vi "Convert Array to image.vi"() -> ()   [LabVIEW 2014]
uses:
  <vilib>/Utility/file.llb/Read From Spreadsheet File (DBL).vi
panel:
  out "Image Out 2":T1(plugin-control)
  out "Picture":picture
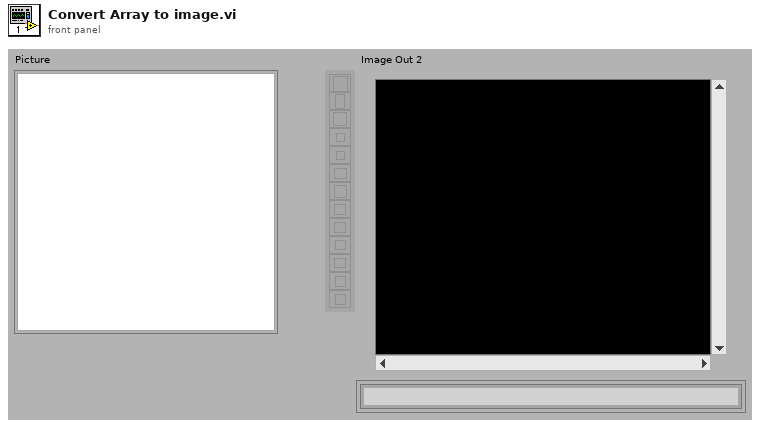
[diagram p1: front panel]
types:
  T1 = typedef "IMAQ Image.ctl" = refnum<image>
  T2 = typedef "imagedata.ctl" = cluster{"image type":i32, "image depth":i32, "image":u8[], "mask":u8[], "colors":u32[], "Rectangle":cluster{"left":i16, "top":i16, "right":i16, "bottom":i16}}
  T3 = cluster{"Position":cluster{"X":sgl, "Y":sgl}, "Radius":dbl, "Score":dbl}[]
  T4 = cluster{"Corners":cluster{"X":sgl, "Y":sgl}[], "Orientation (degrees)":dbl, "Width":dbl, "Height":dbl, "Score":dbl}[]
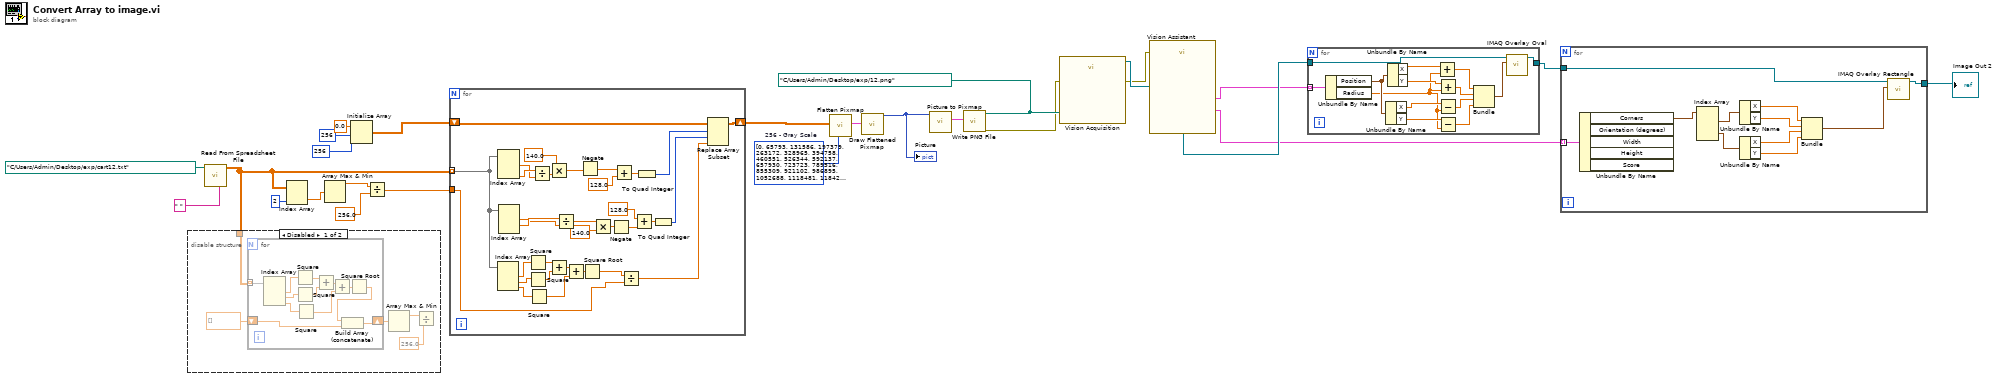
[diagram p0: block diagram]
diagram:
  w12 = path "C:/Users/Admin/Desktop/exp/12.png" ("path to PNG file")
  w15 = u32[] [0, 65793, 131586, 197379, 263172, 328965, 394758, 460551, 526344, 592137, 657930, 723723, 789516, 855309, 921102, 986895, 1052688, 1118481, 1184274, 1250067, 1315860, 1381653, 1447446, 1513239, 1579032, 1644825, 1710618, 1776411, 1842204, 1907997, 1973790, 2039583, 2105376, 2171169, 2236962, 2302755, 2368548, 2434341, 2500134, 2565927, 2631720, 2697513, 2763306, 2829099, 2894892, 2960685, 3026478, 3092271, 3158064, 3223857, 3289650, 3355443, 3421236, 3487029, 3552822, 3618615, 3684408, 3750201, 3815994, 3881787, 3947580, 4013373, 4079166, 4144959, 4210752, 4276545, 4342338, 4408131, 4473924, 4539717, 4605510, 4671303, 4737096, 4802889, 4868682, 4934475, 5000268, 5066061, 5131854, 5197647, 5263440, 5329233, 5395026, 5460819, 5526612, 5592405, 5658198, 5723991, 5789784, 5855577, 5921370, 5987163, 6052956, 6118749, 6184542, 6250335, 6316128, 6381921, 6447714, 6513507, 6579300, 6645093, 6710886, 6776679, 6842472, 6908265, 6974058, 7039851, 7105644, 7171437, 7237230, 7303023, 7368816, 7434609, 7500402, 7566195, 7631988, 7697781, 7763574, 7829367, 7895160, 7960953, 8026746, 8092539, 8158332, 8224125, 8289918, 8355711, 8421504, 8487297, 8553090, 8618883, 8684676, 8750469, 8816262, 8882055, 8947848, 9013641, 9079434, 9145227, 9211020, 9276813, 9342606, 9408399, 9474192, 9539985, 9605778, 9671571, 9737364, 9803157, 9868950, 9934743, 10000536, 10066329, 10132122, 10197915, 10263708, 10329501, 10395294, 10461087, 10526880, 10592673, 10658466, 10724259, 10790052, 10855845, 10921638, 10987431, 11053224, 11119017, 11184810, 11250603, 11316396, 11382189, 11447982, 11513775, 11579568, 11645361, 11711154, 11776947, 11842740, 11908533, 11974326, 12040119, 12105912, 12171705, 12237498, 12303291, 12369084, 12434877, 12500670, 12566463, 12632256, 12698049, 12763842, 12829635, 12895428, 12961221, 13027014, 13092807, 13158600, 13224393, 13290186, 13355979, 13421772, 13487565, 13553358, 13619151, 13684944, 13750737, 13816530, 13882323, 13948116, 14013909, 14079702, 14145495, 14211288, 14277081, 14342874, 14408667, 14474460, 14540253, 14606046, 14671839, 14737632, 14803425, 14869218, 14935011, 15000804, 15066597, 15132390, 15198183, 15263976, 15329769, 15395562, 15461355, 15527148, 15592941, 15658734, 15724527, 15790320, 15856113, 15921906, 15987699, 16053492, 16119285, 16185078, 16250871, 16316664, 16382457, 16448250, 16514043, 16579836, 16645629, 16711422, 16777215]  # 256 - Gray Scale
  n1 = call-poly <vilib>:"Read From Spreadsheet File.vi"("delimiter (\\t)"=" " ("delimiter (\\t)"), "file path (dialog if empty)"=path "C:/Users/Admin/Desktop/exp/cart12.txt") -> ("all rows"=w4:dbl[][])  [unwired: 5 in, 4 out]
  n2 = disable-structure shown="Disabled" {
    disable-tunnel: w4 -> [w31 _]
    frame Disabled {
      n3 = for {
        tunnel: w31 -> [w35] mode=indexing
        shift-right: [w34] -> w27
        shift-left: dbl[] [] -> [w32]
        n4 = Index Array(array=w35) -> (element #1=w43:dbl, element #2=w42:dbl, element #3=w37:dbl)  [unwired: 3 in]
        n5 = Square(x=w43) -> (x^2=w41:dbl)
        n6 = Square(x=w42) -> (x^2=w40:dbl)
        n7 = Square(x=w37) -> (x^2=w36:dbl)
        n8 = Add(x=w41, y=w40) -> (x+y=w39:dbl)
        n9 = Add(x=w39, y=w36) -> (x+y=w38:dbl)
        n10 = Square Root(x=w38) -> (sqrt(x)=w33:dbl)
        n11 = Build Array (concatenate)(w33, w32) -> (w34:dbl[])
      }
      n12 = Array Max & Min(array=w27) -> (max value=w29:dbl)  [unwired: 3 out]
      n13 = Divide(x=w29, y=256.0) -> ()  [unwired: 1 out]
    }
    frame Enabled {
    }
  }
  n14 = Index Array(array=w4, index (col)=2 ("disabled index (col)")) -> (element=w19:dbl[])  [unwired: 1 in]
  n15 = Array Max & Min(array=w19) -> (max value=w18:dbl)  [unwired: 3 out]
  n16 = Initialize Array(0.0 ("element"), 256 ("dimension size"), 256 ("dimension size")) -> (w21:dbl[][])
  n17 = Divide(x=w18, y=256.0) -> (x/y=w3:dbl)
  n18 = for {
    tunnel: w4 -> [w69] mode=indexing
    shift-right: [w51] -> w16
    shift-left: w21 -> [w50]
    tunnel: w3 -> [w60]
    n19 = Index Array(array=w69) -> (element #1=w75:dbl, element #2=w74:dbl, element #3=w64:dbl)  [unwired: 3 in]
    n20 = Index Array(array=w69) -> (element #1=w56:dbl, element #3=w57:dbl)  [unwired: 3 in, 1 out]
    n21 = Index Array(array=w69) -> (element #1=w54:dbl, element #2=w55:dbl)  [unwired: 3 in, 1 out]
    n22 = Square(x=w75) -> (x^2=w73:dbl)
    n23 = Square(x=w74) -> (x^2=w72:dbl)
    n24 = Square(x=w64) -> (x^2=w63:dbl)
    n25 = Divide(x=w57, y=w56) -> (x/y=w67:dbl)
    n26 = Multiply(x=140.0, y=w67) -> (x*y=w47:dbl)
    n27 = Add(x=w73, y=w72) -> (x+y=w71:dbl)
    n28 = Divide(x=w55, y=w54) -> (x/y=w68:dbl)
    n29 = Add(x=w71, y=w63) -> (x+y=w70:dbl)
    n30 = Negate(x=w47) -> (-x=w46:dbl)
    n31 = Square Root(x=w70) -> (sqrt(x)=w61:dbl)
    n32 = Multiply(x=w68, y=140.0) -> (x*y=w45:dbl)
    n33 = Negate(x=w45) -> (-x=w44:dbl)
    n34 = Add(x=w46, y=128.0 ("x")) -> (x+y=w48:dbl)
    n35 = Divide(x=w61, y=w60) -> (x/y=w62:dbl)
    n36 = Add(x=128.0 ("y"), y=w44) -> (x+y=w49:dbl)
    n37 = To Quad Integer(1:w48) -> (0:w59:i64)
    n38 = To Quad Integer(1:w49) -> (0:w58:i64)
    n39 = Replace Array Subset(array=w50, new element=w62, index (row)=w59, index (col)=w58) -> (w51:dbl[][])
  }
  n40 = call <vilib>:"Flatten Pixmap.vi"("colors"=w15, "8-bit pixmap"=w16) -> ("image data"=w13:T2)  [unwired: 9 in]
  n41 = call <vilib>:"Draw Flattened Pixmap.vi"("image data"=w13) -> ("new picture"=w26:picture)  [unwired: 8 in]
  "Picture" <- w26
  n42 = call <vilib>:"Picture to Pixmap.vi"("picture"=w26) -> ("image data"=w14:T2)  [unwired: 9 in, 1 out]
  n43 = call <vilib>:"Write PNG File.vi"("image data"=w14, "path to PNG file"=w12) -> ("error out"=w2:errorcluster)  [unwired: 8 in, 1 out]
  n44 = call "Vision Acquisition"("Image Path"=w12, "error in"=w2) -> ("Image Out"=w9:T1, "error out"=w1:errorcluster)  [unwired: 24 in]
  n45 = call "Vision Assistant"("Image In"=w9, "error in"=w1) -> ("Image Out"=w11:T1, "Circles (Shape Detection 1)"=w6:T3, "Rectangles (Copy of Shape Detection 1)"=w5:T4)  [unwired: 22 in, 1 out]
  n46 = for {
    tunnel: w11 -> [w89]
    tunnel: [w77] -> w8
    tunnel: w6 -> [w76] mode=indexing
    n47 = Unbundle By Name(w76) -> ("Position"=w86:cluster{"X":sgl, "Y":sgl}, "Radius"=w83:dbl)
    n48 = Unbundle By Name(w86) -> ("X"=w85:sgl, "Y"=w84:sgl)
    n49 = Unbundle By Name(w86) -> ("X"=w88:sgl, "Y"=w87:sgl)
    n50 = Add(x=w88, y=w83) -> (x+y=w79:dbl)
    n51 = Add(x=w87, y=w83) -> (x+y=w82:dbl)
    n52 = Subtract(x=w85, y=w83) -> (x-y=w81:dbl)
    n53 = Subtract(x=w84, y=w83) -> (x-y=w80:dbl)
    n54 = Bundle(w79, w82, w81, w80) -> (w78:cluster{dbl, dbl, dbl, dbl})  [unwired: 1 in]
    n55 = call "IMAQ Overlay Oval"("Bounding Rectangle"=w78, "Image"=w89) -> ("Image Out"=w77:T1)  [unwired: 8 in, 1 out]
  }
  n56 = for {
    tunnel: w8 -> [w100]
    tunnel: [w99] -> w10
    tunnel: w5 -> [w90] mode=indexing
    n57 = Unbundle By Name(w90) -> ("Corners"=w98:cluster{"X":sgl, "Y":sgl}[])  [unwired: 4 out]
    n58 = Index Array(array=w98) -> (element #1=w97:cluster{"X":sgl, "Y":sgl}, element #3=w96:cluster{"X":sgl, "Y":sgl})  [unwired: 4 in, 2 out]
    n59 = Unbundle By Name(w97) -> ("X"=w93:sgl, "Y"=w95:sgl)
    n60 = Unbundle By Name(w96) -> ("X"=w94:sgl, "Y"=w92:sgl)
    n61 = Bundle("X"=w93, "Y"=w95, "X"=w94, "Y"=w92) -> (w91:cluster{"X":sgl, "Y":sgl, "X":sgl, "Y":sgl})  [unwired: 1 in]
    n62 = call "IMAQ Overlay Rectangle"("Rectangle"=w91, "Image"=w100) -> ("Image Out"=w99:T1)  [unwired: 8 in, 1 out]
  }
  "Image Out 2" <- w10
